vi "NOx Data.vi"() -> ()   [LabVIEW 2016]
uses:
  <vilib>/Powertrain Controls/Device Drivers/DCM/Tools/RT/NOx Data.ctl
  <vilib>/Powertrain Controls/Device Drivers/DCM/Tools/RT/DCM - RT - Tools.lvlib
panel:
  in  "NOx Data":T2 {"NOx Sensor Data 2"."Sensor Supply Status" items=["NOT IN RANGE", "SUPPLY IN RANGE", "ERROR", "NOT AVAILABLE"]; "NOx Sensor Data 2"."Sensor Temperature Status" items=["NOT AT TEMPERATURE"=0, "AT TEMPERATURE"=4, "ERROR"=8, "NOT AVAILABLE"=12]; "NOx Sensor Data 2"."NOx Signal Status" items=["NOT VALID"=0, "VALID"=16, "ERROR"=32, "NOT AVAILABLE"=48]; "NOx Sensor Data 2"."O2 Signal Status" items=["NOT VALID"=0, "VALID"=64, "ERROR"=128, "NOT AVAILABLE"=192]; "NOx Sensor Data 2"."Heater Mode Status" items=["AUTO MODE"=0, "HEATUP SLOPE 3 OR 4"=32, "HEATUP SLOPE 1 OR 2"=64, "HEATER OFF / PREHEAT"=96]; "NOx Sensor Data 2"."Heater Circuit Status" items=["OPEN WIRE"=3, "SHORT CIRCUIT"=5, "NO ERROR"=31]; "NOx Sensor Data 2"."NOx Circuit Status" items=["OPEN WIRE"=3, "SHORT CIRCUIT"=5, "NO ERROR"=31]; "NOx Sensor Data 2"."O2 Circuit Status" items=["OPEN WIRE"=3, "SHORT CIRCUIT"=5, "NO ERROR"=31]; "NOx Sensor Data 2"."O2 [%}" format="%#_3p"; "NOx Sensor Data 2"."NOx [ppm]" format="%#_3p"; "NOx Sensor Data"."Sensor Supply Status" items=["NOT IN RANGE", "SUPPLY IN RANGE", "ERROR", "NOT AVAILABLE"]; "NOx Sensor Data"."Sensor Temperature Status" items=["NOT AT TEMPERATURE"=0, "AT TEMPERATURE"=4, "ERROR"=8, "NOT AVAILABLE"=12]; "NOx Sensor Data"."NOx Signal Status" items=["NOT VALID"=0, "VALID"=16, "ERROR"=32, "NOT AVAILABLE"=48]; "NOx Sensor Data"."O2 Signal Status" items=["NOT VALID"=0, "VALID"=64, "ERROR"=128, "NOT AVAILABLE"=192]; "NOx Sensor Data"."Heater Mode Status" items=["AUTO MODE"=0, "HEATUP SLOPE 3 OR 4"=32, "HEATUP SLOPE 1 OR 2"=64, "HEATER OFF / PREHEAT"=96]; "NOx Sensor Data"."Heater Circuit Status" items=["OPEN WIRE"=3, "SHORT CIRCUIT"=5, "NO ERROR"=31]; "NOx Sensor Data"."NOx Circuit Status" items=["OPEN WIRE"=3, "SHORT CIRCUIT"=5, "NO ERROR"=31]; "NOx Sensor Data"."O2 Circuit Status" items=["OPEN WIRE"=3, "SHORT CIRCUIT"=5, "NO ERROR"=31]; "NOx Sensor Data"."O2 [%}" format="%#_3p"; "NOx Sensor Data"."NOx [ppm]" format="%#_3p"}
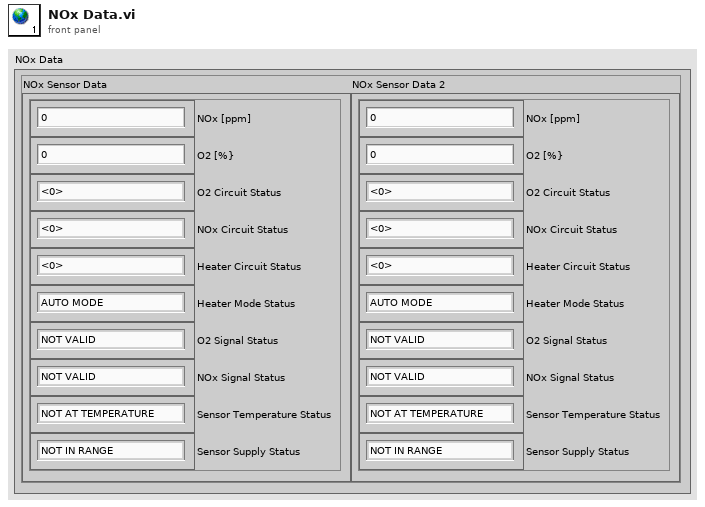
[diagram p1: front panel]
types:
  T1 = typedef "DCM - RT - Tools.lvlib/NOx Data.ctl" = cluster{"NOx [ppm]":sgl, "O2 [%}":sgl, "O2 Circuit Status":u8, "NOx Circuit Status":u8, "Heater Circuit Status":u8, "Heater Mode Status":u8, "O2 Signal Status":u8, "NOx Signal Status":u8, "Sensor Temperature Status":u8, "Sensor Supply Status":u8}
  T2 = cluster{"NOx Sensor Data":T1, "NOx Sensor Data 2":T1}
diagram:
